vi "Teleop.vi"(10 "Match Info":T1={"Autonomous Elapsed Seconds"=0.0, "TeleOp Elapsed Seconds"=0.0, "Disabled Elapsed Seconds"=0.0, "Visited Autonomous"=FALSE, "Visited TeleOp"=FALSE, "Visited Disabled"=FALSE, "Autonomous Settings"={"Autonomous Style"=enum."Independent", "VI Refnum"=refnum}}, 11 "Call Context":T2) -> ()   [LabVIEW 2016]
doc: "This VI is called for each TeleOp packet received from the DS where the robot is not disabled. It is often used to read from the joysticks and update I/O or to update setpoints for timed control loops. It should complete and return within 20 milliseconds or it may miss DS packets."
uses:
  <vilib>/Rock Robotics/WPI/DriverStation/WPI_DriverStationDerivedRobotMode.ctl
  <vilib>/Rock Robotics/WPI/DriverStation/WPI_DriverStationMatch Info.ctl
  SUPPORT/Joystick Axes Enum.ctl
  <vilib>/Rock Robotics/WPI/Utilities/WPI_GetSetVariantRefNum.vi
  <vilib>/Rock Robotics/Network Tables/NT Write Boolean Array.vi
  <vilib>/Rock Robotics/Network Tables/NT Write Numeric Array.vi
  <vilib>/Rock Robotics/WPI/RobotDrive/WPI_RobotDriveArcadeDrive_Standard(NoSaturation).vi
  <vilib>/Rock Robotics/WPI/Ultrasonic/WPI_SonarMB1010AnalogRefNum Registry Get.vi
  <vilib>/Rock Robotics/WPI/Ultrasonic/WPI_SonarMB1010AnalogGetRange.vi
  <vilib>/Rock Robotics/Network Tables/NT Write Number.vi
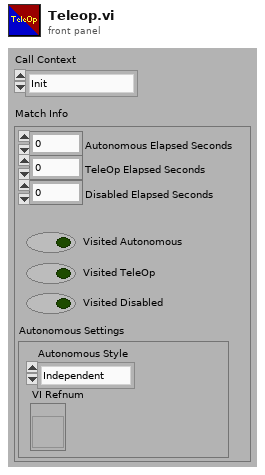
[diagram p1: front panel]
types:
  T1 = typedef "WPI_DriverStationMatch Info.ctl" = cluster{"Autonomous Elapsed Seconds":dbl, "TeleOp Elapsed Seconds":dbl, "Disabled Elapsed Seconds":dbl, "Visited Autonomous":bool, "Visited TeleOp":bool, "Visited Disabled":bool, "Autonomous Settings":cluster{"Autonomous Style":enum16{"Iterative", "Independent"}, "VI Refnum":refnum<vi>}}
  T2 = typedef "WPI_DriverStationDerivedRobotMode.ctl" = enum16{"Init", "Execute", "Stop"}
  T3 = typedef "Joystick Axes Enum.ctl" = enum16{"X-Axis", "Y-Axis", "Z-Axis", "Slider (Throttle)"}
  T4 = typedef "WPI_SonarMB1010AnalogDeviceRef.ctl" = cluster{"AIDeviceRef":T5, "Scaling factor (V/in)":dbl, "Average Bits":u8}
  T5 = typedef "WPI_AnalogChannelDevRef.ctl" = cluster{"DevStatus":errorcluster, "Analog Channel":T6}
  T6 = typedef "FPGA_AIChannel.ctl" = enum8{"AI 0", "AI 1", "AI 2", "AI 3", "AI MXP 0", "AI MXP 1", "AI MXP 2", "AI MXP 3", "Invalid"}
  T7 = typedef "WPI_JoystickDevRef.ctl" = cluster{"Device":T8}
  T8 = typedef "WPI_JoystickDeviceEnum.ctl" = enum16{"USB 0", "USB 1", "USB 2", "USB 3", "USB 4", "USB 5"}
  T9 = typedef "WPI_RobotDriveDevRef.ctl" = cluster{"DevStatus":errorcluster, "Motors[]":T10[], "Square Inputs":bool, "Max Output":dbl}
  T10 = typedef "WPI_MotorControlDeviceRef.ctl" = cluster{"DeviceStatus":errorcluster, "Type":T11, "PWM":cluster{"PWM Channel":T12, "DeadBand":T13}, "CAN":cluster{"Device Number":u8, "SetOutput VI Ref":variant, "GetOutput VI Ref":variant, "Enable VI Ref":variant, "Disable VI Ref":variant, "Data":variant}, "Invert":bool}
  T11 = typedef "WPI_MotorControlType.ctl" = enum16{"PWM", "CAN"}
  T12 = typedef "FPGA_DIOPWMChannel.ctl" = enum8{"PWM 0", "PWM 1", "PWM 2", "PWM 3", "PWM 4", "PWM 5", "PWM 6", "PWM 7", "PWM 8", "PWM 9", "PWM MXP 0", "PWM MXP 1", "PWM MXP 2", "PWM MXP 3", "PWM MXP 4", "PWM MXP 5", "PWM MXP 6", "PWM MXP 7", "PWM MXP 8", "PWM MXP 9", "Invalid"}
  T13 = typedef "WPI_PWMDeadband.ctl" = cluster{"Name":string, "maxPositivePwm":i32, "minPositivePwm":i32, "centerPwm":i32, "maxNegativePwm":i32, "minNegativePwm":i32, "angularRange":u16}
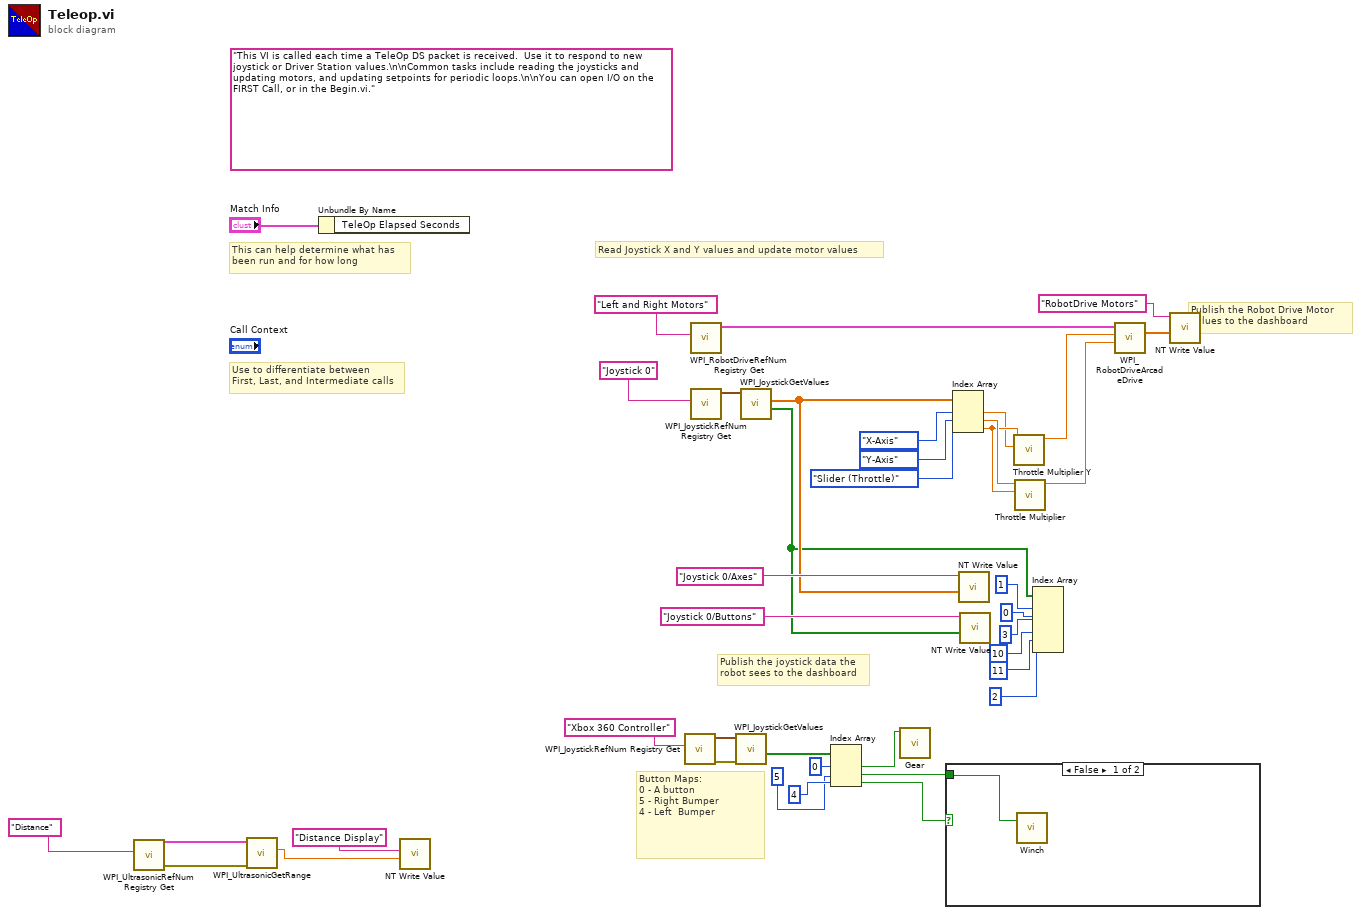
[diagram p0: block diagram]
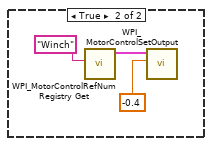
[diagram p2: hidden frame]
diagram:
  (unwired) "This VI is called each time a TeleOp DS packet is received.  Use it to respond to new joystick or Driver Station values.\n\nCommon tasks include reading the joysticks and updating motors, and updating setpoints for periodic loops.\n\nYou can open I/O on the FIRST Call, or in the Begin.vi."
  # "Button Maps:\n0 - A button\n5 - Right Bumper\n4 - Left  Bumper"
  # "Publish the Robot Drive Motor\nvalues to the dashboard"
  # "Publish the joystick data the\nrobot sees to the dashboard"
  # "Use to differentiate between\nFirst, Last, and Intermediate calls"
  # "This can help determine what has\nbeen run and for how long"
  # "Read Joystick X and Y values and update motor values"
  n1 = call-poly <vilib>:"WPI_UltrasonicRefNum Registry Get.vi"("refnum name"="Distance") -> ("error out"=w25:errorcluster, "SonarMB1010AnalogDevRef"=w26:T4)  [unwired: 9 in]
  n2 = call-poly <vilib>:"WPI_UltrasonicGetRange.vi"("error in"=w25, "SonarMB1010AnalogDevRef"=w26) -> ("Distance"=w24:dbl)  [unwired: 7 in, 2 out]
  n3 = Unbundle By Name("Match Info") -> ()  [unwired: 1 out]
  n4 = call-poly <vilib>:"NT Write Value.vi"("Numeric"=w24, "Name"="Distance Display") -> ()  [unwired: 9 in, 1 out]
  n5 = call <vilib>:"WPI_JoystickRefNum Registry Get.vi"("refnum name"="Xbox 360 Controller") -> ("error out"=w18:errorcluster, "JoystickDevRef"=w17:T7)  [unwired: 1 in, 8 out]
  n6 = call <vilib>:"WPI_RobotDriveRefNum Registry Get.vi"("refnum name"="Left and Right Motors") -> ("RobotDriveDevRef"=w4:T9)  [unwired: 1 in, 9 out]
  n7 = call <vilib>:"WPI_JoystickRefNum Registry Get.vi"("refnum name"="Joystick 0") -> ("JoystickDevRef"=w37:T7)  [unwired: 1 in, 9 out]
  n8 = call <vilib>:"WPI_JoystickGetValues.vi"("error in (no error)"=w18, "JoystickDevRef"=w17) -> ("Buttons"=w15:bool[])  [unwired: 5 in, 4 out]
  n9 = call <vilib>:"WPI_JoystickGetValues.vi"("JoystickDevRef"=w37) -> ("Buttons"=w33:bool[], "Axes"=w34:dbl[])  [unwired: 6 in, 3 out]
  n10 = Index Array(array=w15, index #1=0 ("index"), index #2=5 ("index"), index #3=4 ("index")) -> (element #1=w1:bool, element #2=w8:bool, element #3=w7:bool)
  n11 = call "Gear.vi"("Button 0"=w1) -> ()  [unwired: 9 in]
  n12 = case shown="False" w7 {
    tunnel: w8 -> [w41 _]
    frame False {
      n13 = call "Winch.vi"("Button 0"=w41) -> ()  [unwired: 2 in]
    }
    frame True {
      n14 = call <vilib>:"WPI_MotorControlRefNum Registry Get.vi"("refnum name"="Winch") -> ("MotorControlDevRef"=w43:T10)  [unwired: 9 in, 1 out]
      n15 = call <vilib>:"WPI_MotorControlSetOutput.vi"("Output"=-0.4, "MotorControlDevRef"=w43) -> ()  [unwired: 7 in, 3 out]
    }
  }
  n16 = Index Array(array=w34, index #1=Joystick_Axes_Enum."X-Axis" ("Joystick Axes"), index #2=Joystick_Axes_Enum."Y-Axis" ("Joystick Axes"), index #3=Joystick_Axes_Enum."Slider (Throttle)" ("Joystick Axes")) -> (element #1=w11:dbl, element #2=w13:dbl, element #3=w12:dbl)
  n17 = call-poly <vilib>:"NT Write Value.vi"("Numeric Array"=w34, "Name"="Joystick 0/Axes") -> ()  [unwired: 9 in, 1 out]
  n18 = call-poly <vilib>:"NT Write Value.vi"("Boolean Array"=w33, "Name"="Joystick 0/Buttons") -> ()  [unwired: 9 in, 1 out]
  n19 = call "Throttle Multiplier Y.vi"("Input"=w11, "Slider"=w12) -> ("Output"=w2:dbl)  [unwired: 9 in]
  n20 = call "Throttle Multiplier.vi"("Slider"=w12, "Input"=w13) -> ("Output"=w3:dbl)  [unwired: 9 in]
  n21 = Index Array(array=w33, index #1=1 ("index"), index #2=0 ("index"), index #3=3 ("index"), index #4=10 ("index"), index #5=11 ("index"), index #6=2 ("index")) -> ()  [unwired: 6 out]
  n22 = call-poly <vilib>:"WPI_RobotDriveArcadeDrive.vi"("Y axis value"=w3, "X axis value"=w2, "RobotDriveDevRef"=w4) -> ("Motor Values"=w6:dbl[])  [unwired: 6 in, 2 out]
  n23 = call-poly <vilib>:"NT Write Value.vi"("Numeric Array"=w6, "Name"="RobotDrive Motors") -> ()  [unwired: 9 in, 1 out]
